vi "initiate.vi"(0 "reference in":refnum<class "python.lvclass">, 5 "error in (no error)":errorcluster) -> (14 "reference out":refnum<class "python.lvclass">, 19 "error out":errorcluster)   [LabVIEW 2014, in "python.lvclass"]
uses:
  python.lvclass
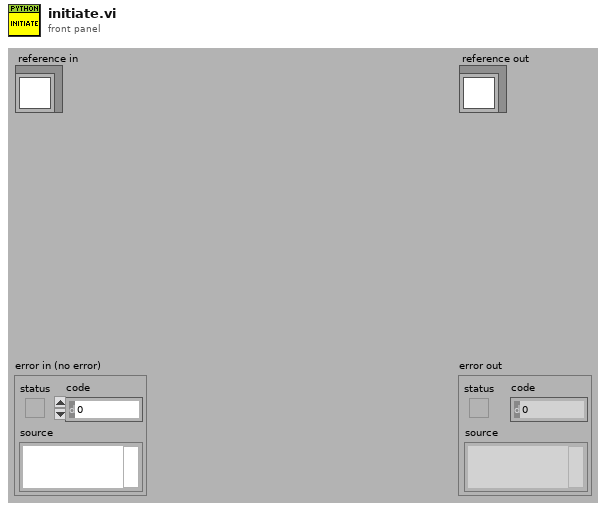
[diagram p1: front panel]
types:
  T1 = typedef "python.lvclass/ObjectAttributesRef.ctl" = refnum<data-value>
  T2 = typedef "python.lvclass/ObjectAttributes.ctl" = cluster{"MyAttribute":dbl, "workingDirectory":path}
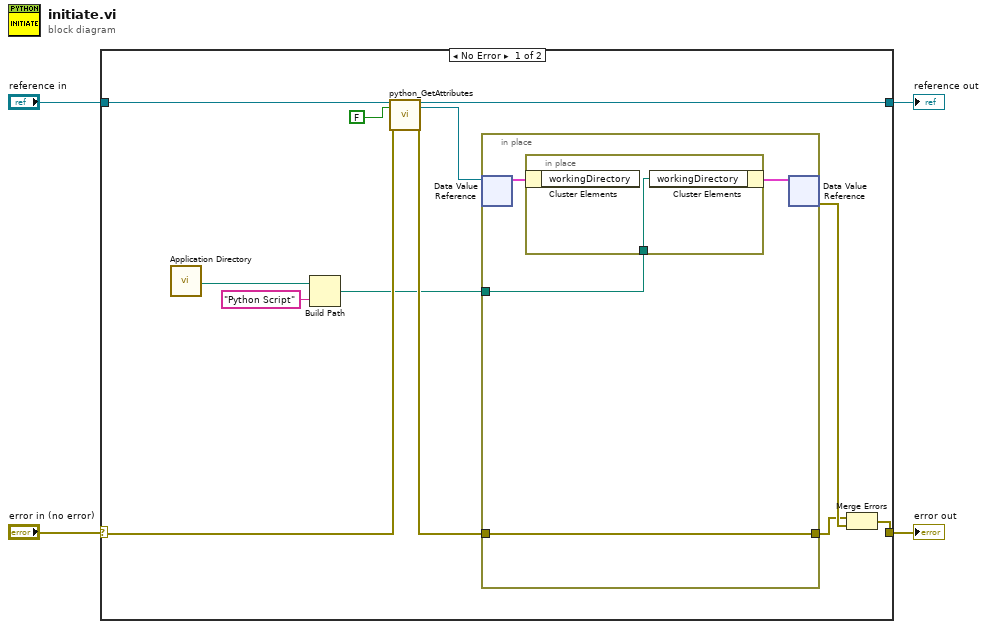
[diagram p0: block diagram]
diagram:
  n1 = case shown="No Error" "error in (no error)" {
    selector: "error in (no error)" -> [w11 w23]
    tunnel: [w16 w23] -> w3
    tunnel: [w9 w22] -> w1
    tunnel: "reference in" -> [w13 w22]
    frame No Error {
      n2 = call <vilib>:"Application Directory.vi"() -> ("Application Directory"=w7:path)
      n3 = Build Path(base path=w7, name or relative path="Python Script") -> (appended path=w5:path)
      n4 = call "python_GetAttributes.vi"("reference in"=w13, "return data? (T)"=FALSE, "error in (no error)"=w11) -> ("reference out"=w9:refnum<class "python.lvclass">, "attributes ref"=w8:T1, "error out"=w10:errorcluster)  [unwired: 13 in, 1 out]
      n5 = in-place {
        in-place-border: w10 -> [w18]
        in-place-border: [w18] -> w14
        in-place-border: w5 -> [w17]
        n6 = in-place-dvr #1(w8) -> (w19:T2)  [unwired: 1 out]
        n7 = in-place {
          in-place-border: w17 -> [w21]
          n8 = in-place-cluster #2(w19) -> ()  [unwired: 1 out]
          n9 = in-place-cluster #2("workingDirectory"=w21) -> (w20:T2)
        }
        n10 = in-place-dvr #1(w20) -> (w15:errorcluster)  [unwired: 1 out]
      }
      n11 = Merge Errors(w14, w15) -> (w16:errorcluster)
    }
    frame Error {
    }
  }
  "error out" <- w3
  "reference out" <- w1
